vi "Matrix_to_Array_of_3d_Arrays.vi"() -> ()   [LabVIEW 2019]
uses:
  <vilib>/Analysis/Matrix/Datatypes/ComplexMatrix.ctl
  <vilib>/Analysis/Matrix/Numeric/Conversions/Matrix To Array - CM.vi
  <vilib>/Analysis/Matrix/NI_Matrix.lvlib
panel:
  out "size(s)":i32[](array[numeric])
  out "output array":cdb[](array[numeric])
  in  "dimension size":i32
  out "Complex 2D Array":cdb[][](array[numeric])
  in  "Complex Matrix":T1
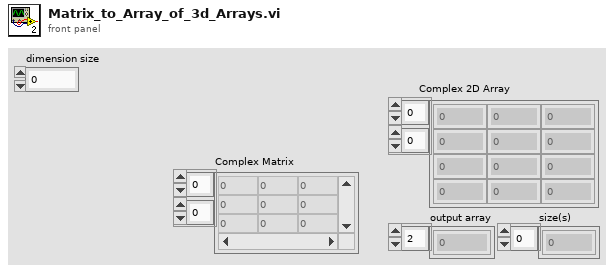
[diagram p1: front panel]
types:
  T1 = typedef "NI_Matrix.lvlib/ComplexMatrix.ctl" = cdb[][]
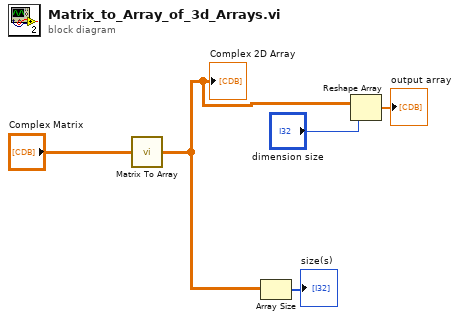
[diagram p0: block diagram]
diagram:
  n1 = call-poly <vilib>:"Matrix To Array.vi"("Complex Matrix"="Complex Matrix") -> ("Complex 2D Array"=w2:cdb[][])
  "Complex 2D Array" <- w2
  n2 = Array Size(array=w2) -> (size(s)=→"size(s)":i32[])
  n3 = Reshape Array(w2, "dimension size") -> (→"output array":cdb[])
